vi "Test API Execution from Test Suite.vi"(8 "error in (no error)":errorcluster, 11 "API Test in":refnum<class "API Test.lvclass">) -> (0 "error out":errorcluster, 3 "API Test out":refnum<class "API Test.lvclass">)   [LabVIEW 2020, in "LUnit Tests.lvlib" / "API Test.lvclass"]
uses:
  API Test.lvclass
  C:/Program Files (x86)/National Instruments/LabVIEW 2020/vi.lib/Astemes/LUnit/Test Case.lvclass
  source/Framework/Test Suite/LUnit Test Suite.lvclass
  Skip First Test Case/Skip First Test Case.lvclass
  C:/Users/anton/Documents/GitHub/LUnit/source/Framework/Test Case/LUnit Test Case.lvclass
  Skip Last Test Case/Skip Last Test Case.lvclass
  source/Framework/Test Suite/LUnit Test Suite.lvclass/LUnit Test Suite.ctl
  source/Framework/Test Case/LUnit Test Case.lvclass/LUnit Test Case.ctl
  source/Framework/Result Classes/Test Suite Result/Test Suite Result.lvclass/Test Suite Result.ctl
  <vilib>/Astemes/LUnit/Test Case.lvclass/Test Case.ctl
  <vilib>/Astemes/LUnit/LUnit Assertion Result.lvclass/LUnit Assertion Result.ctl
  <vilib>/Astemes/LUnit/LUnit Test Case Result.lvclass/LUnit Test Case Result.ctl
  <vilib>/Astemes/LUnit/LUnit Method Result.lvclass/LUnit Method Result.ctl
  source/Framework/Test Case/Public/Accessors/Read Enabled Test Methods.vi
  <vilib>/Astemes/LUnit/Palette/Fail.vi
  <vilib>/Astemes/LUnit/Palette/Pass.vi
  <vilib>/Astemes/LUnit/Set Assertion Type.vi
  <vilib>/Astemes/LUnit/Palette/Pass If Equal.vi/cbf50e99-f124-4847-863a-8e9794d3dede.vi
  <vilib>/Astemes/LUnit/Add test result.vi
  <vilib>/Astemes/LUnit/LUnit Write Passed.vi
  <vilib>/Astemes/LUnit/LUnit Write Message.vi
  <vilib>/Astemes/LUnit/LUnit Write Description.vi
  <vilib>/Astemes/LUnit/LUnit Write Assertion Type.vi
  <vilib>/Astemes/LUnit/Compare Variants.vi
  <vilib>/Astemes/LUnit/Describe Comparison.vi
  <vilib>/Astemes/LUnit/LUnit Record Assertion Result.vi
  <vilib>/Astemes/LUnit/Variant to string.vi
  <vilib>/Astemes/LUnit/LUnit Aggregate Assertion Results.vi
  <vilib>/Astemes/LUnit/Assertion Result/LUnit Read Status.vi
  <vilib>/Astemes/LUnit/LUnit Read Message.vi
  <vilib>/Astemes/LUnit/LUnit Read Description.vi
  <vilib>/Astemes/LUnit/Method Result/LUnit Merge Status.vi
  <vilib>/Astemes/LUnit/LUnit Concatenate result strings.vi
  <vilib>/Utility/Data Type/Get Type Information.vi
  <vilib>/Utility/LVClass/Get LV Class Name.vi
  <vilib>/Astemes/LUnit/LUnit Assertion Result.lvclass
  API Test.lvclass/API Test.ctl
  source/Framework/Execution API/Execution API.lvclass
  <vilib>/Astemes/LUnit/Test Case.lvclass
  source/Framework/Result Classes/Test Suite Result/Test Suite Result.lvclass
  C:/Users/anton/Documents/GitHub/LUnit/tests/API Test/API Test.lvclass
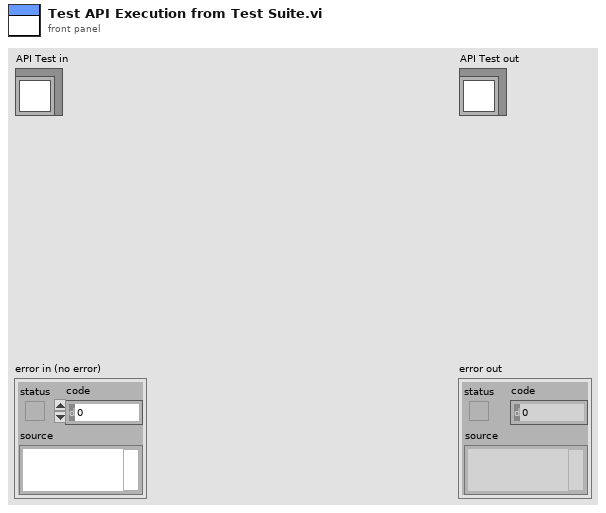
[diagram p1: front panel]
types:
  T1 = cluster{"Event Registration Refnum":refnum<event-registration>, "Event Registration Refnum":refnum<event-registration>}
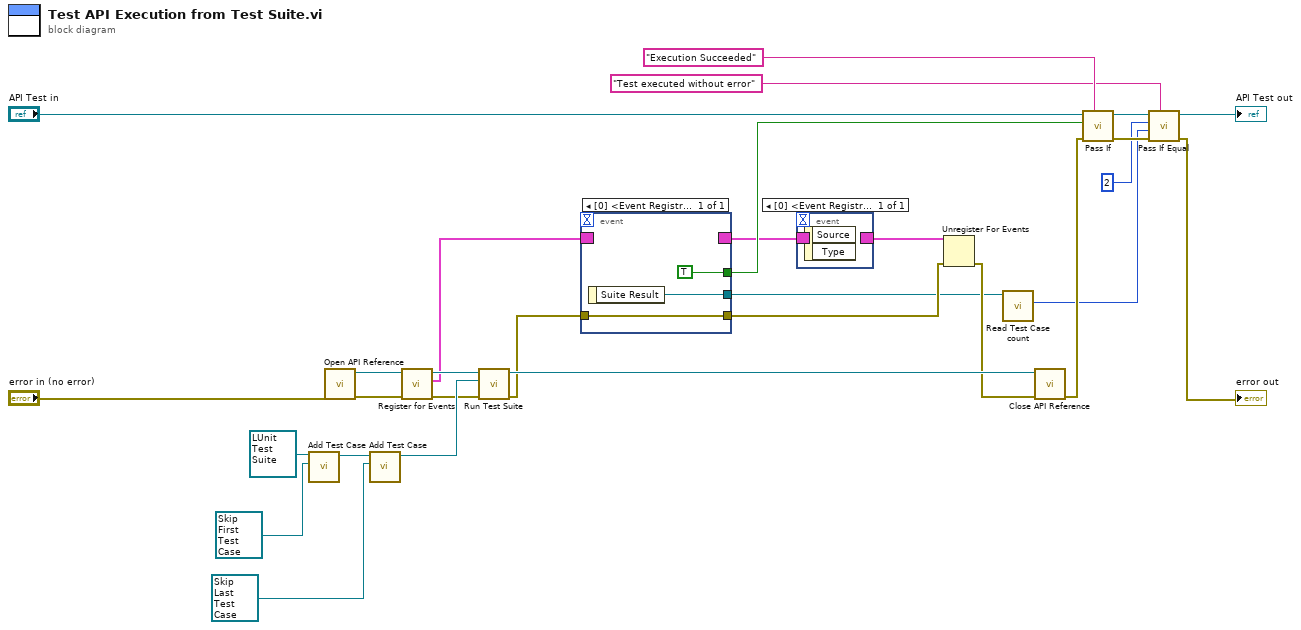
[diagram p0: block diagram]
diagram:
  n1 = call "Add Test Case.vi"("Test Case to add"=refnum<class "Skip First Test Case.lvclass"> refnum ("Skip First Test Case.lvclass"), "Test Suite In"=refnum<class "LUnit Test Suite.lvclass"> refnum) -> ("Test Suite Out"=w16:refnum<class "LUnit Test Suite.lvclass">)  [unwired: 8 in, 1 out]
  n2 = call "Open API Reference.vi"("error in (no error)"="error in (no error)") -> ("error out"=w18:errorcluster, "Execution API out"=w3:refnum<class "Execution API.lvclass">)  [unwired: 9 in]
  n3 = call "Add Test Case.vi"("Test Case to add"=refnum<class "Skip Last Test Case.lvclass"> refnum ("Skip Last Test Case.lvclass"), "Test Suite In"=w16) -> ("Test Suite Out"=w15:refnum<class "LUnit Test Suite.lvclass">)  [unwired: 8 in, 1 out]
  n4 = call "Register for Events.vi"("error in (no error)"=w18, "Execution API In"=w3) -> ("error out"=w4:errorcluster, "Result Events Registration"=w1:T1, "Execution API Out"=w2:refnum<class "Execution API.lvclass">)  [unwired: 7 in]
  n5 = call "Run Test Suite.vi"("error in (no error)"=w4, "Test Case"=w15, "Execution API In"=w2) -> ("error out"=w19:errorcluster, "Execution API Out"=w20:refnum<class "Execution API.lvclass">)  [unwired: 7 in]
  n6 = event shown="[0] <Event Registration Refnum.Suite Result>: User Event" {
    selector: w1 -> [_]
    dyn-events: [_] -> w6
    timeout: _ -> [_]
    tunnel: [TRUE] -> w24
    tunnel: [w31] -> w13
    tunnel: w19 -> [w31]
    tunnel: [w30] -> w12
    event User Event {
      n7 = event-data() -> ("Suite Result"=w30:refnum<class "Test Suite Result.lvclass">)  [unwired: 1 in]
    }
  }
  n8 = event shown="[0] <Event Registration Refnum.Test Completed>: User Event" {
    selector: w6 -> [_]
    dyn-events: [_] -> w5
    timeout: _ -> [_]
    event User Event {
      n9 = event-data() -> ()  [unwired: 1 in, 2 out]
    }
  }
  n10 = Unregister For Events(event registration refnum=w5, error in=w13) -> (error out=w14:errorcluster)
  n11 = call "Read Test Case count.vi"("Test Suite Result In"=w12) -> ("Test Case count"=w10:i32)  [unwired: 9 in, 1 out]
  n12 = call "Close API Reference.vi"("error in (no error)"=w14, "Execution API in"=w20) -> ("error out"=w11:errorcluster)  [unwired: 9 in]
  n13 = call <vilib>:"Pass If.vi"("Description"="Execution Succeeded", "error in (no error)"=w11, "Pass?"=w24, "LUnit Test Case In"="API Test in") -> ("error out"=w25:errorcluster, "LUnit Test Case Out"=w26:refnum<class "API Test.lvclass">)  [unwired: 6 in]
  n14 = call <vilib>:"Pass If Equal.vi"("Description"="Test executed without error", "error in (no error)"=w25, "Actual"=w10, "Expected"=2 ("Test Case count"), "LUnit Test Case In"=w26) -> ("error out"=→"error out":errorcluster, "LUnit Test Case Out"=→"API Test out":refnum<class "API Test.lvclass">)  [unwired: 5 in]
